vi "FrameTrigger6601.vi"(5 "pulse polarity (high:0)":enum16{"high pulse ", "low pulse"}(ring), 7 "Machine Type":enum16{"Hitachi", "B&K 3535", "B&K Hawk"}(ring), 8 "gate edge":T1(ring), 9 "Counter Arm edge":T2(ring)) -> (1 "error out":errorcluster, 2 "task out":refnum<k21>)   [LabVIEW 2022 SP3]
doc: "Configures a counter to generate a single, delayed TTL pulse on its OUT pin. The signal is created by decrementing the counter twice, first for the delay to the pulse (called phase 1), then for the pulse itself (phase 2). The VI selects the highest resolution timebase for the counter to achieve the desired characteristics. You can optionally gate or trigger the operation with a signal on the counter's GATE pin. Call the Counter Start VI to start the pulse or enable it to be gated."
uses:
  <vilib>/DAQmx/create/channels.llb/DAQmx Create Channel (CO-Pulse Generation-Ticks).vi
  <vilib>/DAQmx/configure/trigger.llb/DAQmx Start Trigger (Digital Edge).vi
  <resource>/objmgr/daqmx.rc
panel:
  in  "error in (no error)":errorcluster
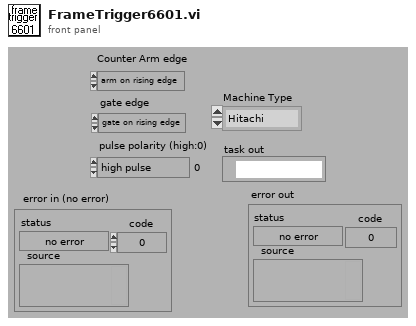
[diagram p1: front panel]
types:
  T1 = enum16{"gate on rising edge", "gate on falling edge"}
  T2 = enum16{"arm on rising edge", "arm on falling edge"}
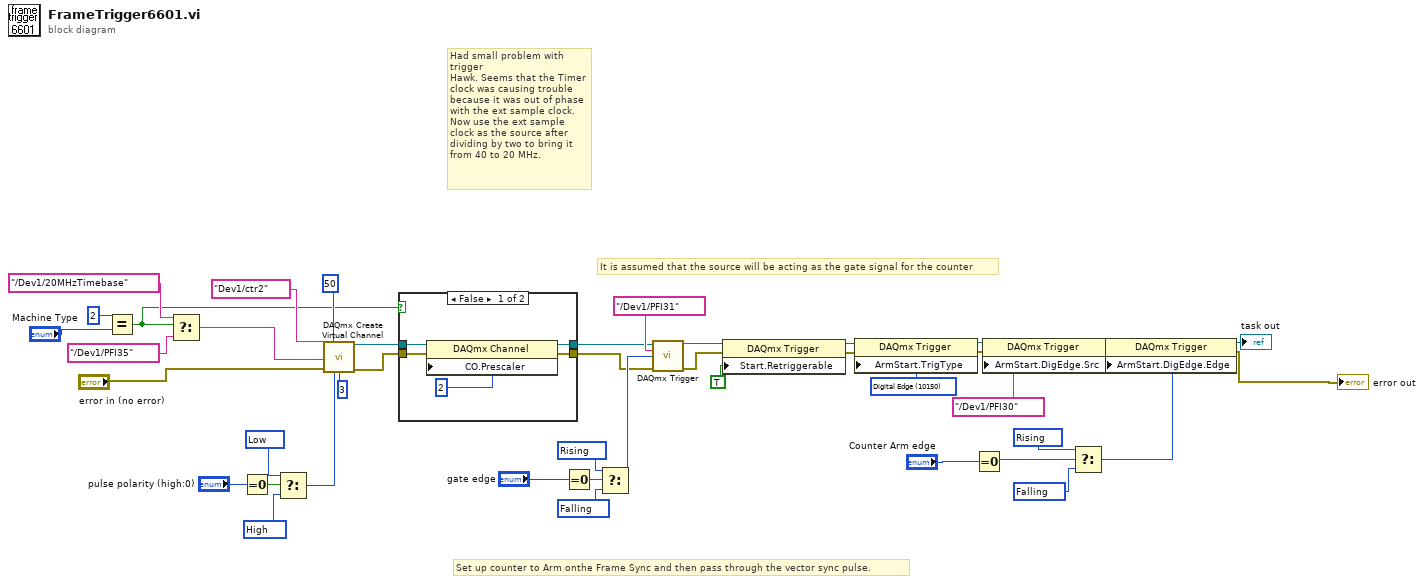
[diagram p0: block diagram]
diagram:
  w1 = 10192 items=["High"=10192, "Low"=10214] ("idle state")
  w2 = 10214 items=["High"=10192, "Low"=10214] ("idle state")
  w21 = 10171 items=["Rising"=10280, "Falling"=10171] ("edge")
  w22 = 10280 items=["Rising"=10280, "Falling"=10171] ("edge")
  w24 = 10150 items=["Digital Edge"=10150, "None"=10230] ("ArmStart.TrigType")
  w26 = 10171 items=["Rising"=10280, "Falling"=10171] ("ArmStart.DigEdge.Edge")
  w27 = 10280 items=["Rising"=10280, "Falling"=10171] ("ArmStart.DigEdge.Edge")
  # "It is assumed that the source will be acting as the gate signal for the counter"
  # "Had small problem with trigger\nHawk. Seems that the Timer clock was causing trouble because it was out of phase with the ext sample clock. Now use the ext sample clock as the source after dividing by two to bring it from 40 to 20 MHz."
  # "Set up counter to Arm onthe Frame Sync and then pass through the vector sync pulse."
  n1 = Equal?(x=2, y="Machine Type") -> (x = y?=w3:bool)
  n2 = Select(t=tag "/Dev1/20MHzTimebase" ("source of ticks"), s=w3, f=tag "/Dev1/PFI35" ("source of ticks")) -> (s? t:f=w6:tag)
  n3 = Equal To 0?(x="pulse polarity (high:0)") -> (x = 0?=w17:bool)
  n4 = Select(t=w2, s=w17, f=w1) -> (s? t:f=w16:i32)
  n5 = call-poly <vilib>:"DAQmx Create Virtual Channel.vi"("high ticks"=50, "counter"=tag "Dev1/ctr2", "source of ticks"=w6, "error in"="error in (no error)", "idle state"=w16, "initial delay"=3) -> ("task out"=w5:refnum<k21>, "error out"=w4:errorcluster)  [unwired: 3 in, 5 out]
  n6 = case shown="False" w3 {
    tunnel: [w48 w50] -> w14
    tunnel: [w47 w49] -> w13
    tunnel: w5 -> [w46 w50]
    tunnel: w4 -> [w45 w49]
    frame False {
      n7 = property class="DAQmx Channel"(reference=w46, error in=w45, "CO.Prescaler"=2) -> (reference out=w48:refnum<k21>, error out=w47:errorcluster)
    }
    frame True {
    }
  }
  n8 = Equal To 0?(x="gate edge") -> (x = 0?=w23:bool)
  n9 = Select(t=w22, s=w23, f=w21) -> (s? t:f=w20:i32)
  n10 = call-poly <vilib>:"DAQmx Trigger.vi"("task/channels in"=w14, "source"=tag "/Dev1/PFI31", "edge"=w20, "error in"=w13) -> ("task out"=w33:refnum<k21>, "error out"=w19:errorcluster)  [unwired: 10 out]
  n11 = property class="DAQmx Trigger"(reference=w33, error in=w19, "Start.Retriggerable"=TRUE) -> (reference out=w32:refnum<k21>, error out=w31:errorcluster)
  n12 = property class="DAQmx Trigger"(reference=w32, error in=w31, "ArmStart.TrigType"=w24) -> (reference out=w30:refnum<k21>, error out=w29:errorcluster)
  n13 = Equal To 0?(x="Counter Arm edge") -> (x = 0?=w25:bool)
  n14 = property class="DAQmx Trigger"(reference=w30, error in=w29, "ArmStart.DigEdge.Src"=tag "/Dev1/PFI30") -> (reference out=w35:refnum<k21>, error out=w34:errorcluster)
  n15 = Select(t=w27, s=w25, f=w26) -> (s? t:f=w28:i32)
  n16 = property class="DAQmx Trigger"(reference=w35, error in=w34, "ArmStart.DigEdge.Edge"=w28) -> (reference out=→"task out":refnum<k21>, error out=→"error out":errorcluster)
